vi "2001_FireAtNoonEveryDay.vi"(8 "error in (no error)":errorcluster) -> (0 "error out":errorcluster)   [LabVIEW 2013]
uses:
  source/Cron.Jenkins/Cron.Jenkins.lvclass/Cron.Jenkins.ctl
  source/Cron.Jenkins/Write Job Name.vi
  <vilib>/addons/_JKI Toolkits/Caraya/classes/Assert/Assert True.vi
  source/Cron/Create Cron Expression.vi
  source/Cron/Compute Next Cron.vi
  source/Cron.Jenkins/Cron.Jenkins.lvclass
  <vilib>/addons/_JKI Toolkits/Caraya/classes/Test/Test.lvclass
  <vilib>/addons/_JKI Toolkits/Caraya/classes/Assert/Assert.lvclass
  source/openCron.lvlib
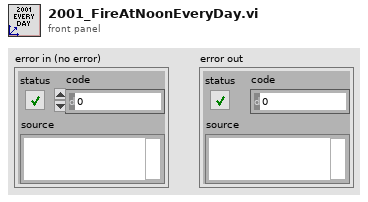
[diagram p1: front panel]
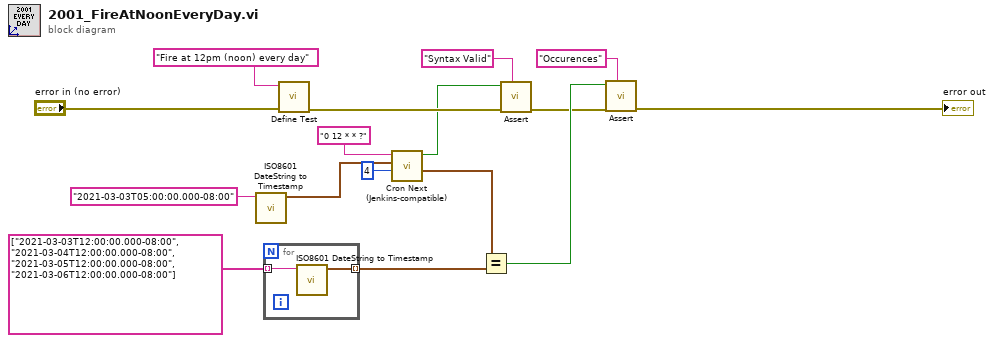
[diagram p0: block diagram]
diagram:
  n1 = call <vilib>:"ISO8601 DateString to Timestamp.vi"("ISO8601 Date String"="2021-03-03T05:00:00.000-08:00" ("Expression")) -> ("Timestamp"=w3:timestamp)  [unwired: 8 in, 2 out]
  n2 = for {
    tunnel: string[] ["2021-03-03T12:00:00.000-08:00", "2021-03-04T12:00:00.000-08:00", "2021-03-05T12:00:00.000-08:00", "2021-03-06T12:00:00.000-08:00"] -> [w18] mode=indexing
    tunnel: [w17] -> w1 mode=indexing
    n3 = call <vilib>:"ISO8601 DateString to Timestamp.vi"("ISO8601 Date String"=w18) -> ("Timestamp"=w17:timestamp)  [unwired: 8 in, 2 out]
  }
  n4 = call <vilib>:"Define Test.vi"("error in (no error)"="error in (no error)", "Label (VI Title)"="Fire at 12pm (noon) every day") -> ("error out"=w10:errorcluster)  [unwired: 8 in, 1 out]
  n5 = call "Cron Next (Jenkins-compatible).vi"("Nb Occurences (min: 1)"=u16 4, "Reference timestamp (Now)"=w3, "Cron Expression"="0 12 * * ?" ("Expression")) -> ("Occurences"=w6:timestamp[], "syntax valid?"=w5:bool)  [unwired: 6 in, 1 out]
  n6 = Equal?(x=w6, y=w1) -> (x = y?=w14:bool)
  n7 = call-poly <vilib>:"Assert.vi"("Label"="Syntax Valid" ("Label (VI Title)"), "error in (no error)"=w10, "True?"=w5) -> ("error out"=w13:errorcluster)  [unwired: 7 in, 1 out]
  n8 = call-poly <vilib>:"Assert.vi"("Label"="Occurences" ("Label (VI Title)"), "error in (no error)"=w13, "True?"=w14) -> ("error out"=→"error out":errorcluster)  [unwired: 7 in, 1 out]
